vi "RestoreROI.vi"(11 "Image In":T1) -> (3 "Image Out":T1)   [LabVIEW 2015]
uses:
  <vilib>/vision/Image Controls.llb/IMAQ Image.ctl
  LiveImage_Global.vi
  AcquisitionGlobals.vi
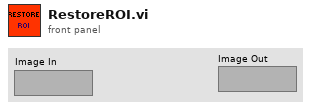
[diagram p1: front panel]
types:
  T1 = typedef "IMAQ Image.ctl" = refnum<image>
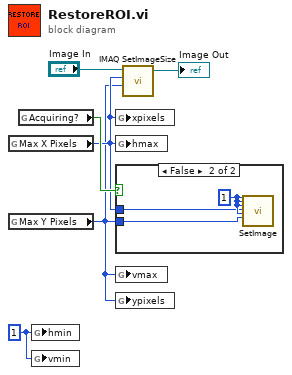
[diagram p0: block diagram]
diagram:
  w6 = 1
  n1 = global read "LiveImage_Global.vi" "Max X Pixels"() -> (w4:i32)
  n2 = global read "LiveImage_Global.vi" "Max Y Pixels"() -> (w3:i32)
  n3 = global read "AcquisitionGlobals.vi" "Acquiring?"() -> (w5:bool)
  n4 = global write "LiveImage_Global.vi" "hmin"(w6) -> ()
  n5 = global write "LiveImage_Global.vi" "vmin"(w6) -> ()
  n6 = global write "LiveImage_Global.vi" "xpixels"(w4) -> ()
  n7 = global write "LiveImage_Global.vi" "hmax"(w4) -> ()
  n8 = case shown="False" w5 {
    tunnel: w4 -> [_ w8]
    tunnel: w3 -> [_ w7]
    frame True {
    }
    frame False {
      w9 = 1 ("hbin")
      n9 = call <userlib>:"SetImage.vi"("hbin"=w9, "vbin"=w9, "hstart"=w9, "hend"=w8, "vstart"=w9, "vend"=w7) -> ()  [unwired: 20 in, 2 out]
    }
  }
  n10 = global write "LiveImage_Global.vi" "vmax"(w3) -> ()
  n11 = global write "LiveImage_Global.vi" "ypixels"(w3) -> ()
  n12 = call "IMAQ SetImageSize"("Y Resolution"=w3, "X Resolution"=w4, "Image"="Image In") -> ("Image Out"=→"Image Out":T1)  [unwired: 2 in, 1 out]
